vi "NT Write Variant.vi"(4 "options":T1={"Send All"=FALSE, "Keep Duplicates"=FALSE, "rate (hz)"=10}, 6 "timestamp":u64, 8 "error in":errorcluster, 9 "variant":variant, 11 "name":string="Variant") -> (0 "error out":errorcluster)   [LabVIEW 2025]
doc: "Write the variant to the named topic."
uses:
  <vilib>/Rock Robotics/Network Tables/NT PublishOptions.ctl
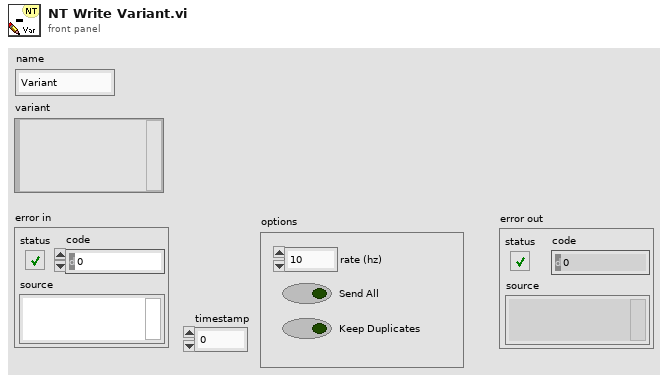
[diagram p1: front panel]
types:
  T1 = typedef "NT PublishOptions.ctl" = cluster{"Send All":bool, "Keep Duplicates":bool, "rate (hz)":u64}
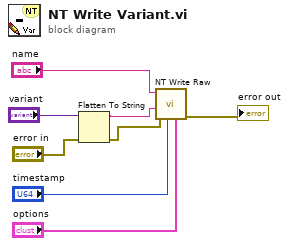
[diagram p0: block diagram]
diagram:
  n1 = Flatten To String(anything="variant", error in (no error)="error in") -> (data string=w6:string, error out=w4:errorcluster)  [unwired: 2 in, 1 out]
  n2 = call <vilib>:"NT Write Raw.vi"("options"="options", "timestamp"="timestamp", "error in"=w4, "value"=w6, "name"="name") -> ("error out"=→"error out":errorcluster)  [unwired: 6 in]
